vi "W vs Z main4c.vi"() -> ()   [LabVIEW 2012]
panel:
  out "FWHM4":dbl format="%.5f"
  out "min w4":dbl format="%.5f"
  out "min  z4":dbl format="%.2f"
  out "contains\nwaist? 4":bool
  in  "lens focal length 4":dbl=-250.0 format="%.3f"
  in  "lens focal length 3":dbl=500.0 format="%.3f"
  in  "FWHM(T)?":bool
  out "contains\nwaist? 1":bool
  out "contains\nwaist? 3":bool
  out "contains\nwaist? 2":bool
  out "FWHM1":dbl format="%.5f"
  out "FWHM3":dbl format="%.5f"
  out "FWHM2":dbl format="%.5f"
  out "Cursor List":T1(array[cluster]) {"Location"."Y" format="%.2f"; "Location"."X" format="%.2f"}
  out "Zor FWHM Array 3":dbl[](array[numeric]) format="%.2f"
  out "Z Array 2":dbl[](array[numeric]) format="%.2f"
  out "Z Array":dbl[](array[numeric]) format="%.2f"
  out "w Array 3":dbl[](array[numeric]) format="%.2f"
  out "w Array 2":dbl[](array[numeric]) format="%.4f"
  out "w Array":dbl[](array[numeric]) format="%.2f"
  out "min w1":dbl format="%.5f"
  out "min w3":dbl format="%.5f"
  in  "z stop":dbl=1000.0 format="%.2f"
  in  "lens focal length 2":dbl=-250.0 format="%.3f"
  in  "N steps":i32=500
  in  "lens focal length":dbl=500.0 format="%.3f"
  out "min  z2":dbl format="%.2f"
  out "min z1":dbl format="%.2f"
  out "min Z3":dbl format="%.2f"
  out "min w2":dbl format="%.5f"
  out "Q start":cdb format="%.4f"
  out "W vs Z":cluster{dbl[], dbl[]}[](graph)
  in  "beam radius(w)":dbl=0.6 format="%.4f"
  in  "Radius of Curvature":dbl=inf format="%.2f"
  in  "Wavelength":dbl=0.00035 format="%.6f"
  in  "z start":dbl format="%.2f"
  # "w is the 1/e field radius"
  # "All values are entered in mm"
  # "w x 1.18 to get FWHM of the Intensity"
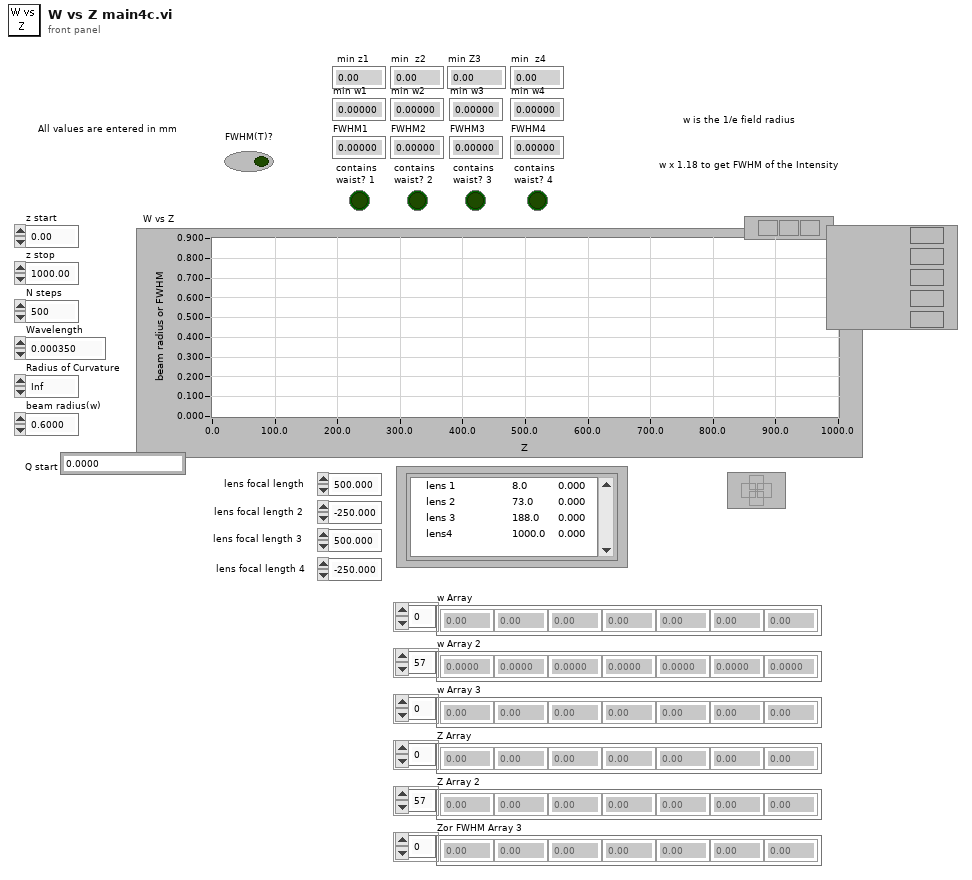
[diagram p1: front panel]
types:
  T1 = cluster{"Name":string, "Color":u32, "Hair Style":u8, "Point Style":u8, "Name Visible":bool, "Trackable":bool, "Lock Style":u32, "Plot Number":u32, "Marker Index":i32, "Location":cluster{"X":dbl, "Y":dbl}}[]
  T2 = cluster{"Name":string, "Color":u32, "Style":u8, "Point Style":u8, "Name Visible":bool, "Allow Drag":bool, "Lock Style":u32, "Plot":u32, "Index":i32, "Position":cluster{"X":dbl, "Y":dbl}}[]
  T3 = cluster{"Name":string, "Color":u32, "Style":u8, "Point Style":u8, "Name Visible":bool, "Allow Drag":bool, "Lock Style":u32, "Plot":u32, "Index":i32, "Position":cluster{"X":dbl, "Y":dbl}}
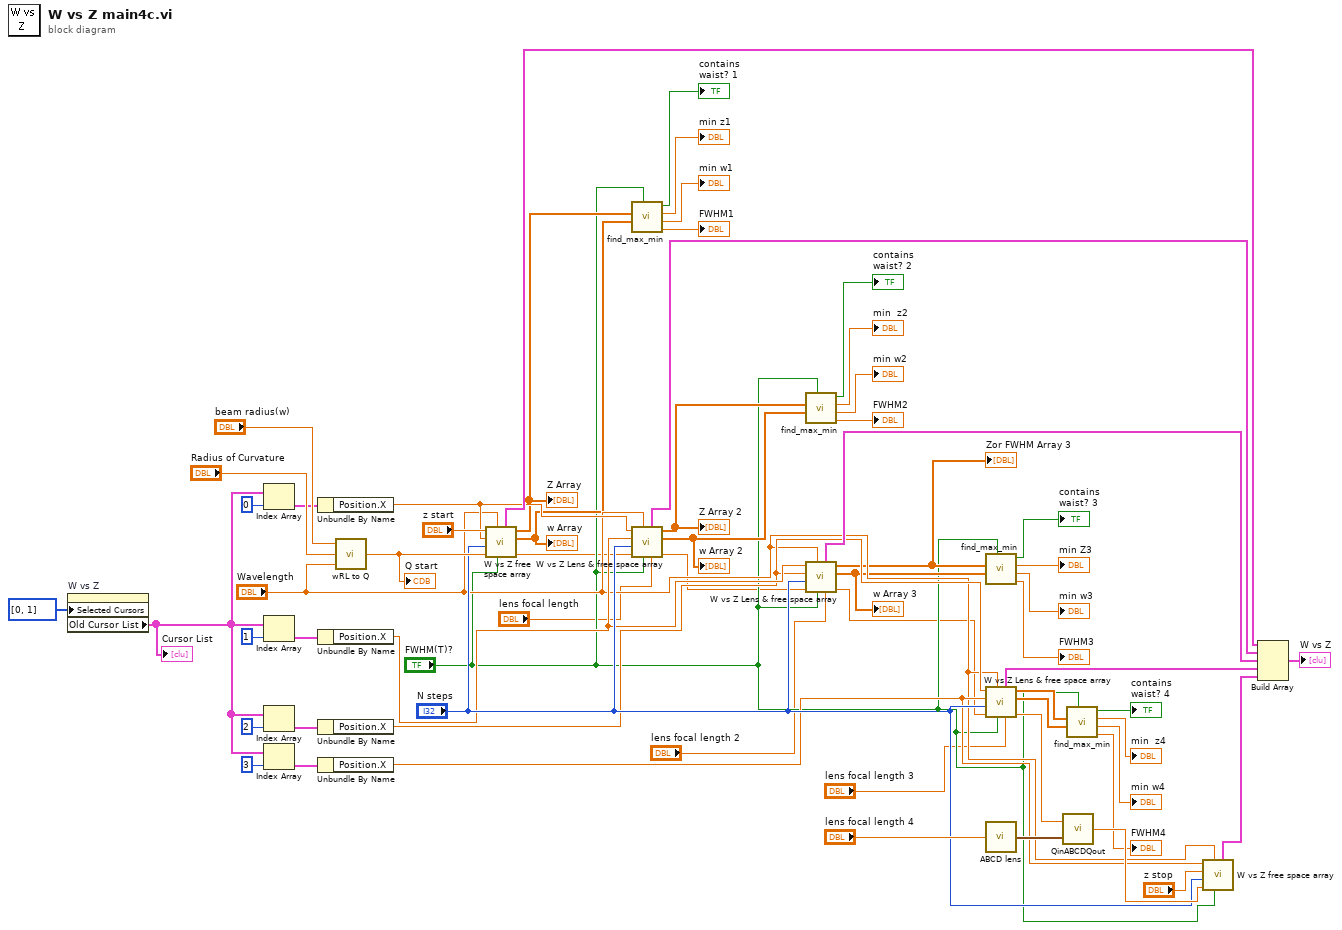
[diagram p0: block diagram]
diagram:
  n1 = property on="W vs Z" class="XYGraph (strict)"("Selected Cursors"=u32[] [0, 1]) -> ("Old Cursor List"=w39:T2)  [unwired: 2 in, 2 out]
  "Cursor List" <- w39
  n2 = Index Array(array=w39, index=0 ("Index")) -> (element=w54:T3)
  n3 = Index Array(array=w39, index=1 ("Index")) -> (element=w52:T3)
  n4 = Index Array(array=w39, index=2 ("Index")) -> (element=w42:T3)
  n5 = Index Array(array=w39, index=3 ("Index")) -> (element=w40:T3)
  n6 = Unbundle By Name(w54) -> ("Position.X"=w38:dbl)
  n7 = Unbundle By Name(w52) -> ("Position.X"=w44:dbl)
  n8 = Unbundle By Name(w42) -> ("Position.X"=w37:dbl)
  n9 = Unbundle By Name(w40) -> ("Position.X"=w36:dbl)
  n10 = call "wRL to Q.vi"("Wavelength"="Wavelength", "Radius of Curvature"="Radius of Curvature", "beam radius(w)"="beam radius(w)") -> ("Q"=w60:cdb)
  "Q start" <- w60
  n11 = call "W vs Z free space array.vi"("FWHM(T)?"="FWHM(T)?", "Wavelength"="Wavelength", "Q start"=w60, "N steps"="N steps", "z stop"=w38, "z start"="z start") -> ("Q out"=w3:cdb, "w/FWHM Array"=w30:dbl[], "Z Array"=w31:dbl[], "W/FWHM vs Z"=w58:cluster{dbl[], dbl[]})  [unwired: 1 out]
  "w Array" <- w30
  "Z Array" <- w31
  n12 = call "find_max_min.vi"("FWHM(T)?"="FWHM(T)?", "w Array"=w30, "z Array"=w31) -> ("FWHM"=→"FWHM1":dbl, "min w"=→"min w1":dbl, "min  z"=→"min z1":dbl, "contains waist?"=→"contains\nwaist? 1":bool)  [unwired: 5 in]
  n13 = call "W vs Z Lens & free space array.vi"("lens focal length"="lens focal length", "FWHM(T)?"="FWHM(T)?", "Wavelength"="Wavelength", "Q in"=w3, "N steps"="N steps", "z stop"=w44, "z start"=w38) -> ("Q out"=w5:cdb, "w/FWHM Array"=w25:dbl[], "Z Array"=w24:dbl[], "W/FWHM vs Z"=w57:cluster{dbl[], dbl[]})  [unwired: 1 out]
  "w Array 2" <- w25
  "Z Array 2" <- w24
  n14 = call "find_max_min.vi"("FWHM(T)?"="FWHM(T)?", "w Array"=w25, "z Array"=w24) -> ("FWHM"=→"FWHM2":dbl, "min w"=→"min w2":dbl, "min  z"=→"min  z2":dbl, "contains waist?"=→"contains\nwaist? 2":bool)  [unwired: 5 in]
  n15 = call "W vs Z Lens & free space array.vi"("lens focal length"="lens focal length 2", "FWHM(T)?"="FWHM(T)?", "Wavelength"="Wavelength", "Q in"=w5, "N steps"="N steps", "z stop"=w37, "z start"=w44) -> ("Q out"=w1:cdb, "w/FWHM Array"=w19:dbl[], "Z Array"=w20:dbl[], "W/FWHM vs Z"=w56:cluster{dbl[], dbl[]})  [unwired: 1 out]
  "w Array 3" <- w19
  "Zor FWHM Array 3" <- w20
  n16 = call "find_max_min.vi"("FWHM(T)?"="FWHM(T)?", "w Array"=w19, "z Array"=w20) -> ("FWHM"=→"FWHM3":dbl, "min w"=→"min w3":dbl, "min  z"=→"min Z3":dbl, "contains waist?"=→"contains\nwaist? 3":bool)  [unwired: 5 in]
  n17 = call "W vs Z Lens & free space array.vi"("lens focal length"="lens focal length 3", "FWHM(T)?"="FWHM(T)?", "Wavelength"="Wavelength", "Q in"=w1, "N steps"="N steps", "z stop"=w36, "z start"=w37) -> ("Q out"=w48:cdb, "w/FWHM Array"=w12:dbl[], "Z Array"=w13:dbl[], "W/FWHM vs Z"=w34:cluster{dbl[], dbl[]})  [unwired: 1 out]
  n18 = call "ABCD lens.vi"("Focal length"="lens focal length 4") -> ("ABCD"=w49:cluster{"A":dbl, "B":dbl, "C":dbl, "D":dbl})
  n19 = call "QinABCDQout.vi"("ABCD"=w49, "Q in"=w48) -> ("Q out"=w47:cdb)
  n20 = call "find_max_min.vi"("FWHM(T)?"="FWHM(T)?", "w Array"=w12, "z Array"=w13) -> ("FWHM"=→"FWHM4":dbl, "min w"=→"min w4":dbl, "min  z"=→"min  z4":dbl, "contains waist?"=→"contains\nwaist? 4":bool)  [unwired: 5 in]
  n21 = call "W vs Z free space array.vi"("FWHM(T)?"="FWHM(T)?", "Wavelength"="Wavelength", "Q start"=w47, "N steps"="N steps", "z stop"="z stop", "z start"=w36) -> ("W/FWHM vs Z"=w33:cluster{dbl[], dbl[]})  [unwired: 4 out]
  n22 = Build Array(w58, w57, w56, w34, w33) -> (→"W vs Z":cluster{dbl[], dbl[]}[])
